vi "SubStage_OpenNewWorkBook.vi"(2 "error in (no error)":errorcluster, 3 "File Path":path, 4 "Excel._Application":refnum<k7>) -> (0 "error out":errorcluster, 1 "Excel._Workbook":refnum<k7>)   [LabVIEW 2015]
doc: "Opens a new WorkBook. Takes an Application Refnum as input."
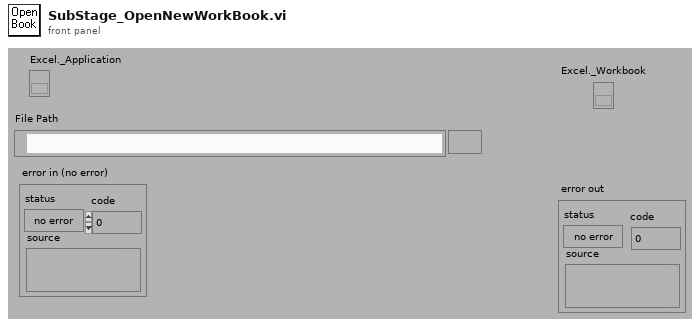
[diagram p1: front panel]
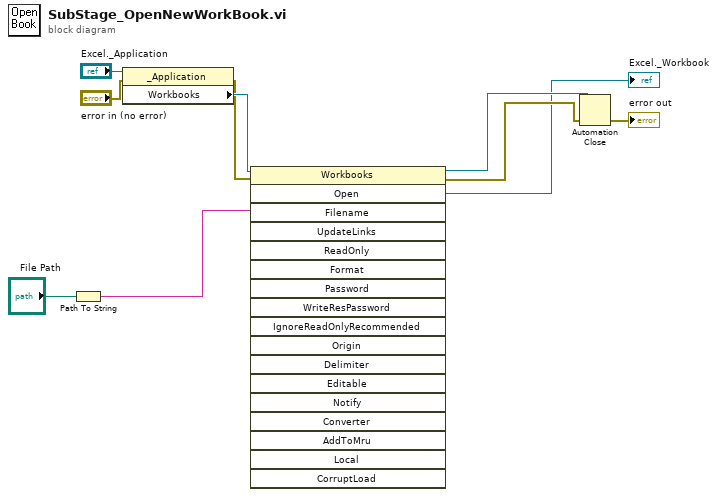
[diagram p0: block diagram]
diagram:
  n1 = Path To String(path="File Path") -> (string=w1:string)
  n2 = property class="_Application"(reference="Excel._Application", error in="error in (no error)") -> (error out=w5:errorcluster, "Workbooks"=w7:refnum<k7>)  [unwired: 1 out]
  n3 = invoke class="Workbooks" method="Open"(reference=w7, error in=w5, "Filename"=w1) -> (reference out=w6:refnum<k7>, error out=w4:errorcluster, "Open"=→"Excel._Workbook":refnum<k7>)  [unwired: 15 in, 15 out]
  n4 = Automation Close(3:w4, 5:w6) -> (0:→"error out":errorcluster)
